vi "获取层次结构.vi"() -> ()   [LabVIEW 2020]
uses:
  <vilib>/Utility/traverseref.llb/TRef TravTarget.ctl
  <vilib>/Utility/traverseref.llb/VI Scripting - Traverse.lvlib
panel:
  out "依赖关系路径":path[](array[path])
  out "数组":string[](array[string])
  out "所有对象[]":string[][](table)
  out "只遍历循环 2":string[][](table)
  out "遍历全部 2":string[][](table)
  in  "Path to Entrance VI":path=path "Test - Using Traverse.vi"
  # "C:\\Users\\Fred\\Desktop\\LabAI\\get_status_code.vi"
  # "C:\\Users\\Fred\\Desktop\\FL62风洞主控软件\\Desktop\\2.4米风洞主控软件20240716\\主程序 - 一键启动-web.vi"
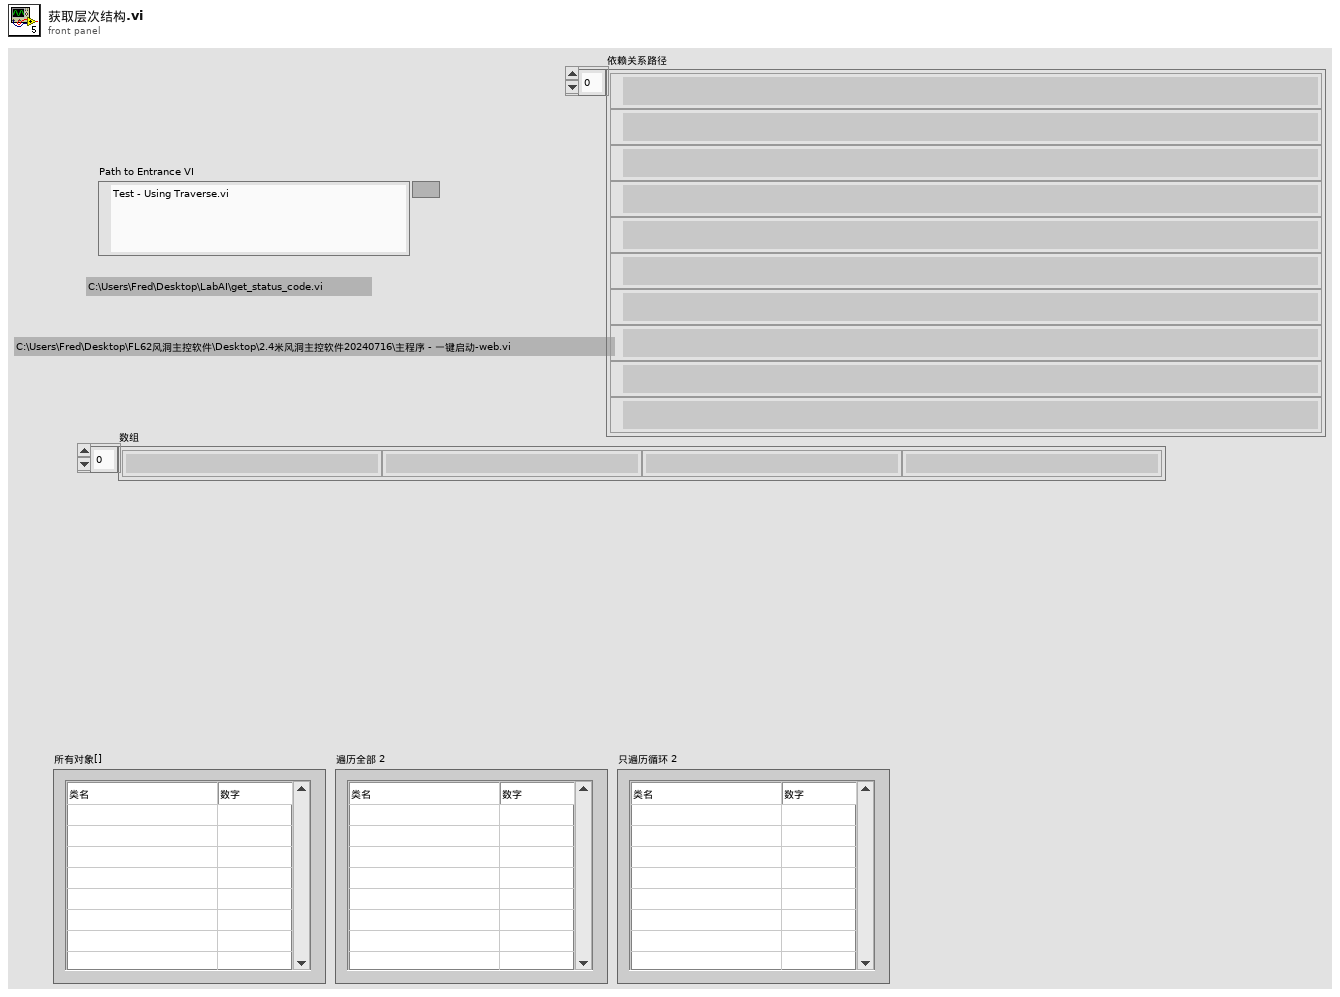
[diagram p1: front panel]
types:
  T1 = typedef "TRef TravTarget.ctl" = enum16{"FP", "BD", "Other"}
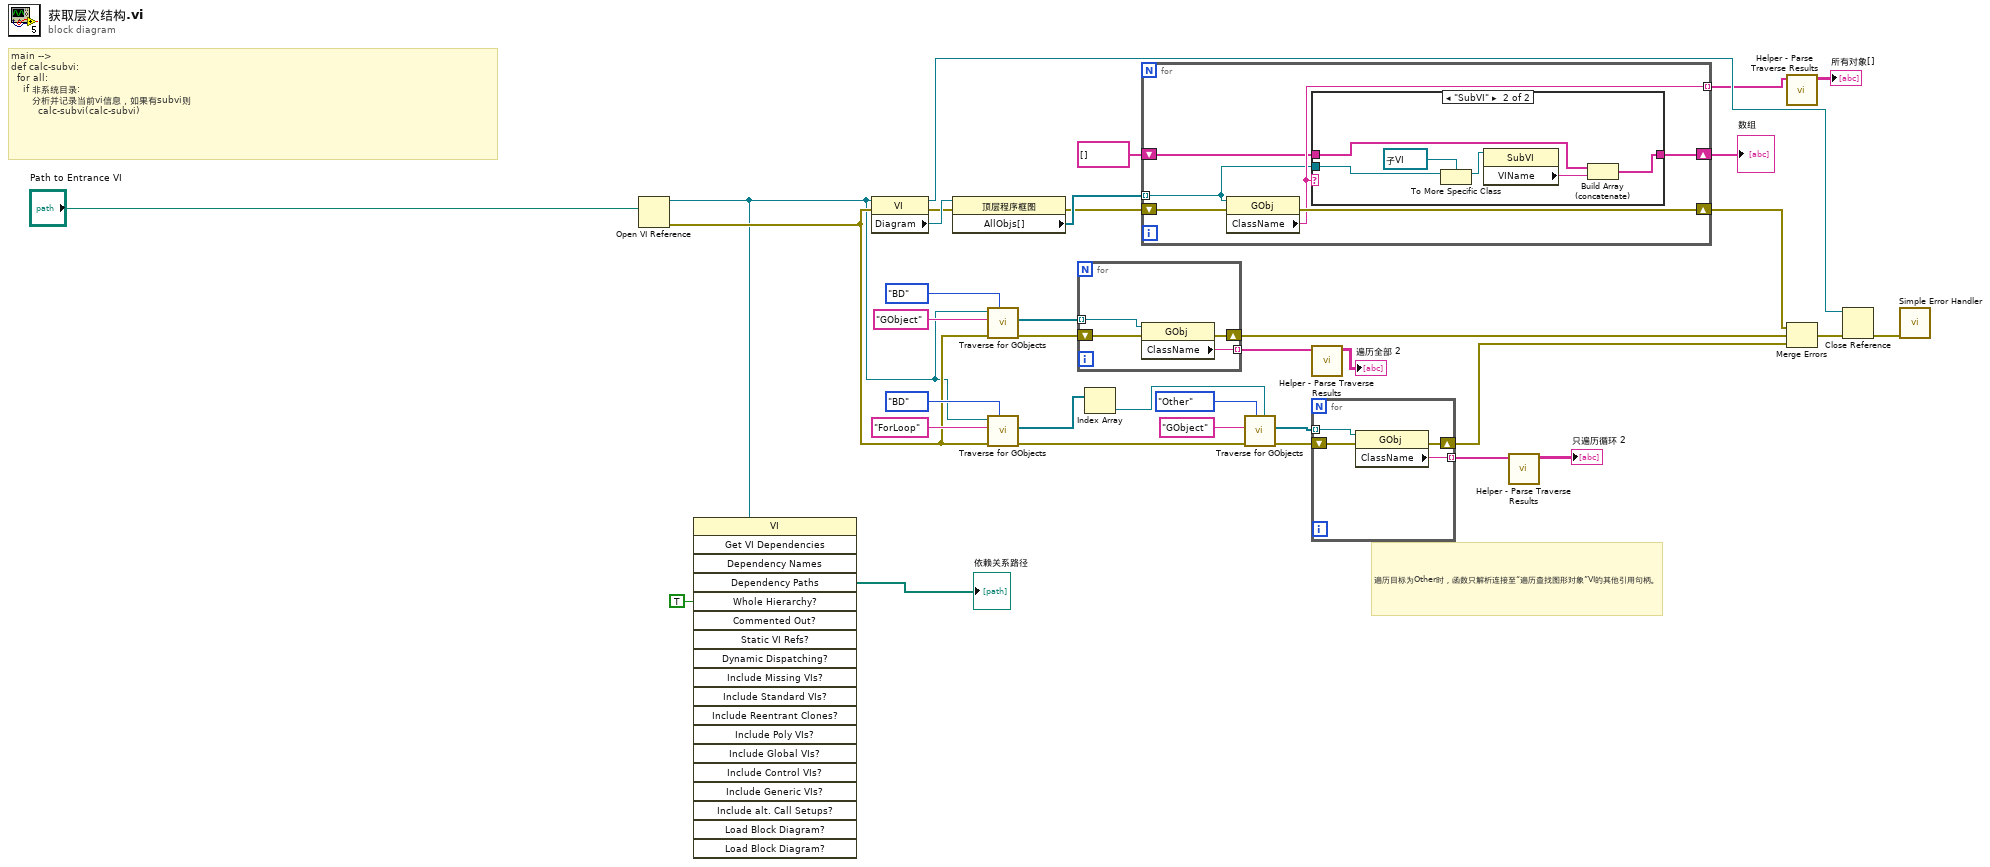
[diagram p0: block diagram]
diagram:
  # "遍历目标为Other时，函数只解析连接至“遍历查找图形对象”VI的其他引用句柄。"
  # "main --> \ndef calc-subvi:\n  for all:\n    if 非系统目录:\n       分析并记录当前vi信息，如果有subvi则\n         calc-subvi(calc-subvi)"
  n1 = Open VI Reference(vi path="Path to Entrance VI") -> (vi reference=w3:refnum<vi>, error out=w28:errorcluster)  [unwired: 5 in]
  n2 = invoke class="VI" method="Get VI Dependencies"(reference=w3, "Whole Hierarchy?"=TRUE ("整个层次结构？")) -> ("Dependency Paths"=→"依赖关系路径":path[])  [unwired: 17 in, 18 out]
  n3 = property class="VI"(reference=w3, error in=w28) -> (reference out=w34:refnum<vi>, error out=w25:errorcluster, "Diagram"=w26:refnum<vi>)
  n4 = property class="顶层程序框图"(reference=w26, error in=w25) -> (error out=w24:errorcluster, "AllObjs[]"=w27:refnum<vi>[])  [unwired: 1 out]
  n5 = call <vilib>:"Traverse for GObjects.vi"("Traverse Target"=TRef_TravTarget."BD", "error in (no error)"=w28, "Class Name"="GObject", "VI Refnum"=w3) -> ("error out"=w17:errorcluster, "References"=w18:refnum<vi>[])  [unwired: 4 in, 2 out]
  n6 = call <vilib>:"Traverse for GObjects.vi"("Traverse Target"=TRef_TravTarget."BD", "error in (no error)"=w28, "Class Name"="ForLoop", "VI Refnum"=w3) -> ("error out"=w30:errorcluster, "References"=w31:refnum<vi>[])  [unwired: 4 in, 2 out]
  n7 = for {
    tunnel: w18 -> [w40] mode=indexing
    tunnel: [w39] -> w15 mode=indexing
    shift-right: [w37] -> w16
    shift-left: w17 -> [w38]
    n8 = property class="GObj"(reference=w40, error in=w38) -> (error out=w37:errorcluster, "ClassName"=w39:string)  [unwired: 1 out]
  }
  n9 = Index Array(array=w31) -> (element=w32:refnum<vi>)  [unwired: 1 in]
  n10 = for {
    tunnel: w27 -> [w43] mode=indexing
    tunnel: [w44] -> w22 mode=indexing
    shift-right: [w45] -> w35
    shift-left: w24 -> [w46]
    shift-right: [w42] -> w4
    shift-left: string[] [] -> [w41]
    n11 = property class="GObj"(reference=w43, error in=w46) -> (error out=w45:errorcluster, "ClassName"=w44:string)  [unwired: 1 out]
    n12 = case shown="\"SubVI\"" w44 {
      tunnel: w43 -> [_ w50]
      tunnel: [w47 w49] -> w42
      tunnel: w41 -> [w47 w48]
      frame "假", Default {
      }
      frame "SubVI" {
        n13 = To More Specific Class(target class=refnum<vi> refnum ("引用"), reference=w50) -> (specific class reference=w53:refnum<vi>)  [unwired: 1 in, 1 out]
        n14 = property class="SubVI"(reference=w53) -> ("VIName"=w52:string)  [unwired: 1 in, 2 out]
        n15 = Build Array (concatenate)(w48, w52) -> (w49:string[])
      }
    }
  }
  "数组" <- w4
  n16 = call <vilib>:"Traverse for GObjects.vi"("Other Refnum"=w32, "Traverse Target"=TRef_TravTarget."Other", "error in (no error)"=w30, "Class Name"="GObject") -> ("error out"=w10:errorcluster, "References"=w9:refnum<vi>[])  [unwired: 4 in, 2 out]
  n17 = call "Helper - Parse Traverse Results.vi"("遍历结果"=w15) -> ("解析结果"=→"遍历全部 2":string[][])  [unwired: 10 in]
  n18 = for {
    tunnel: w9 -> [w57] mode=indexing
    tunnel: [w56] -> w7 mode=indexing
    shift-right: [w54] -> w8
    shift-left: w10 -> [w55]
    n19 = property class="GObj"(reference=w57, error in=w55) -> (error out=w54:errorcluster, "ClassName"=w56:string)  [unwired: 1 out]
  }
  n20 = call "Helper - Parse Traverse Results.vi"("遍历结果"=w7) -> ("解析结果"=→"只遍历循环 2":string[][])  [unwired: 10 in]
  n21 = call "Helper - Parse Traverse Results.vi"("遍历结果"=w22) -> ("解析结果"=→"所有对象[]":string[][])  [unwired: 10 in]
  n22 = Merge Errors(w35, w16, w8) -> (w23:errorcluster)
  n23 = Close Reference(reference=w34, error in (no error)=w23) -> (error out=w36:errorcluster)
  n24 = call <vilib>:"Simple Error Handler.vi"("error in (no error)"=w36) -> ()  [unwired: 4 in, 5 out]
